vi "THz100HzSignauxChemin_SD.vi"(2 "chemin du dossier":path=path "C:/Documents and Settings/radiolyse/Mes documents/data/081023", 3 "nom":string="081023_16:37:04") -> (0 "chemin du fichier RAW":path, 1 "chemin du fichier DAT":path)   [LabVIEW 2015]
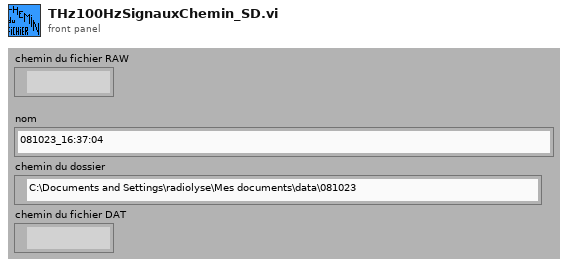
[diagram p1: front panel]
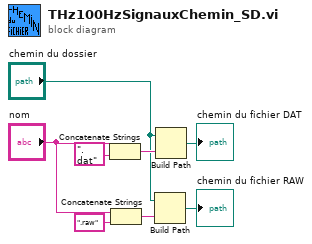
[diagram p0: block diagram]
diagram:
  n1 = Concatenate Strings("nom", ".dat" ("nom ou chemin relatif")) -> (w7:string)
  n2 = Concatenate Strings("nom", ".raw" ("nom ou chemin relatif")) -> (w4:string)
  n3 = Build Path(base path="chemin du dossier", name or relative path=w4) -> (appended path=→"chemin du fichier RAW":path)
  n4 = Build Path(base path="chemin du dossier", name or relative path=w7) -> (appended path=→"chemin du fichier DAT":path)
